vi "Convert to SR Request Enum.vi"(8 "Error In":errorcluster, 11 "SR Status in":string) -> (0 "Error Out":errorcluster)   [LabVIEW 2016, in "Data Operations.lvlib"]
uses:
  Data Operations.lvlib
  Private Controls/SR Status.ctl
  <vilib>/Utility/Data Type/NI_Data Type.lvlib
panel:
  out "Enum Names":string[](array[string])
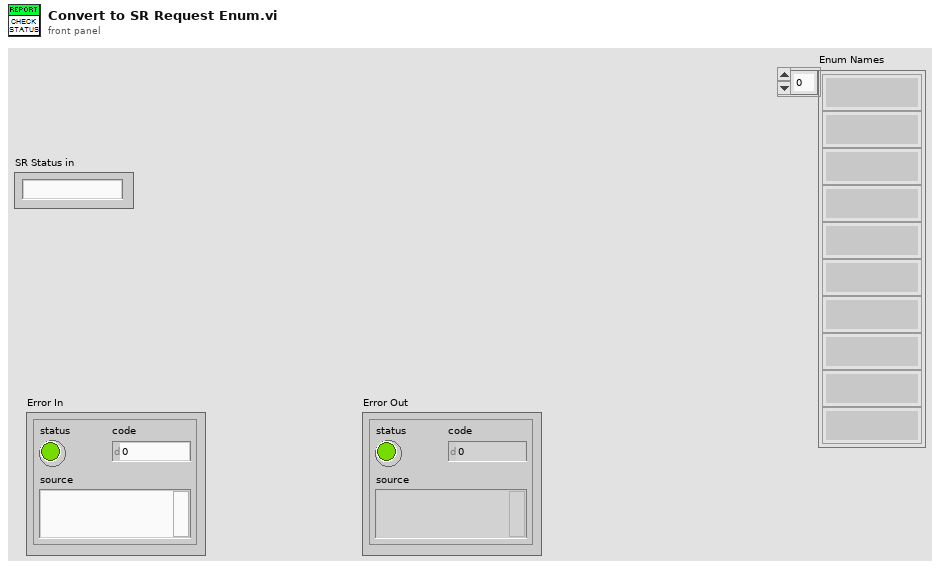
[diagram p1: front panel]
types:
  T1 = typedef "Data Operations.lvlib/SR Status.ctl" = enum16{"IN WORK Wait on Customer", "Presumed Resolved", "Resolved", "IN WORK", "Potentially Resolved", "Open"}
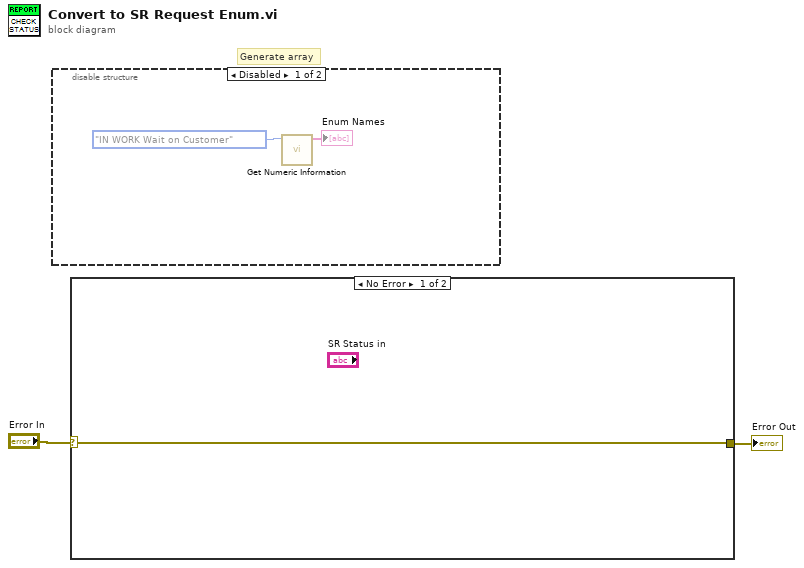
[diagram p0: block diagram]
diagram:
  # "Generate array"
  n1 = disable-structure shown="Disabled" {
    frame Disabled {
      n2 = call <vilib>:"Get Numeric Information.vi"("Variant"=SR_Status."IN WORK Wait on Customer" ("Status")) -> ("Enum Names"=→"Enum Names":string[])  [unwired: 7 in, 3 out]
    }
    frame Enabled {
    }
  }
  n3 = case shown="No Error" "Error In" {
    selector: "Error In" -> [w5 w6]
    tunnel: [w5 w6] -> w1
    frame No Error {
    }
    frame Error {
    }
  }
  "Error Out" <- w1
